vi "Fetch - NT Enum (Index).vi"(7 "PV name":string, 8 "error in":errorcluster, 10 "default index":u16, 11 "Server in":refnum<class "Server.lvclass">) -> (0 "error out":errorcluster, 1 "PV not found?":bool, 2 "index":u16, 3 "Server out":refnum<class "Server.lvclass">, 4 "timestamp":timestamp)   [LabVIEW 2020, in "PV Access.lvlib" / "PVA Server.lvlib" / "Server.lvclass"]
uses:
  Server.lvclass
  Server.lvclass/Server.ctl
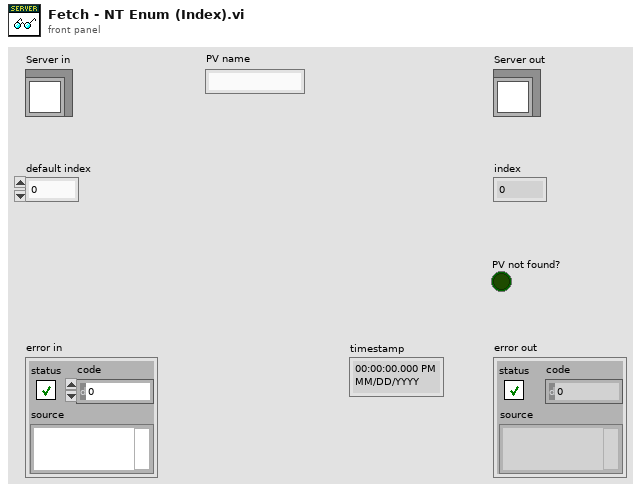
[diagram p1: front panel]
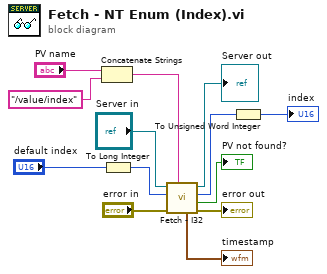
[diagram p0: block diagram]
diagram:
  n1 = Concatenate Strings("PV name", "/value/index") -> (w11:string)
  n2 = To Long Integer(number="default index") -> (32bit integer=w7:i32)
  n3 = call "Fetch - I32.vi"("PV name"=w11, "error in"="error in", "default"=w7, "Server in"="Server in") -> ("error out"=→"error out":errorcluster, "PV not found?"=→"PV not found?":bool, "value"=w6:i32, "Server out"=→"Server out":refnum<class "Server.lvclass">, "timestamp"=→"timestamp":timestamp)  [unwired: 3 in]
  n4 = To Unsigned Word Integer(number=w6) -> (unsigned 16bit integer=→"index":u16)
